vi "Actor Core.vi"(8 "error in":errorcluster, 11 "BrowerController in":refnum<class "BrowerController.lvclass">) -> (0 "error out":errorcluster, 3 "Actor out":refnum<class "Actor.lvclass">)   [LabVIEW 2015, in "BrowerController.lvclass"]
doc: "(<B>Filename</B>: Actor Framework.lvlib:Actor.lvclass:Actor Core.vi)\n\nReceives messages to the actor, reacts to them, and initiates any error handling that may shut the actor down.\n\nDescendant classes may override this VI to append parallel tasks for the actor to complete while it handles messages. Overrides use the Call Parent Method node."
uses:
  BrowerController.lvclass
  <vilib>/ActorFramework/Actor/Actor.lvclass
  Models/BrowerShortcut/BrowerShortcut.lvclass
  Type Definition/Brower UI Refs.ctl
  Models/BrowerTree/BrowerTree.lvclass
  Models/BrowerComponent/BrowerComposite/BrowerComposite.lvclass
  BrowerController.lvclass/BrowerController.ctl
  <vilib>/ActorFramework/Actor/Actor.lvclass/Actor.ctl
  <vilib>/ActorFramework/Message Enqueuer/Message Enqueuer.lvclass/Message Enqueuer.ctl
  Models/BrowerTree/Type Definition/Symbol Index.ctl
  Models/BrowerBuilder/ProjectBuilder/ProjectBuilder.lvclass
  Messages/Add BrowerComponent_Msg/Add BrowerComponent_Msg.lvclass/Add BrowerComponent_Msg.ctl
  Messages/ImportProject_Msg/ImportProject_Msg.lvclass/ImportProject_Msg.ctl
  <vilib>/ActorFramework/Message Enqueuer/Init from Existing Queue.vi
  <vilib>/ActorFramework/Message Enqueuer/Enqueue.vi
  <vilib>/ActorFramework/Message Priority Queue/Priority Enqueue.vi
  <vilib>/ActorFramework/Message Enqueuer/Message Enqueuer.lvclass
  Messages/Add BrowerComponent_Msg/Add BrowerComponent_Msg.lvclass
  Messages/SaveBrowerProject_Msg/SaveBrowerProject_Msg.lvclass
  Messages/ImportProject_Msg/ImportProject_Msg.lvclass
panel:
  out "Value":string
  out "ItemTag":string
  in  "String: BrowerMenu Selection":string
  in  "Tree: Brower":string(tree)
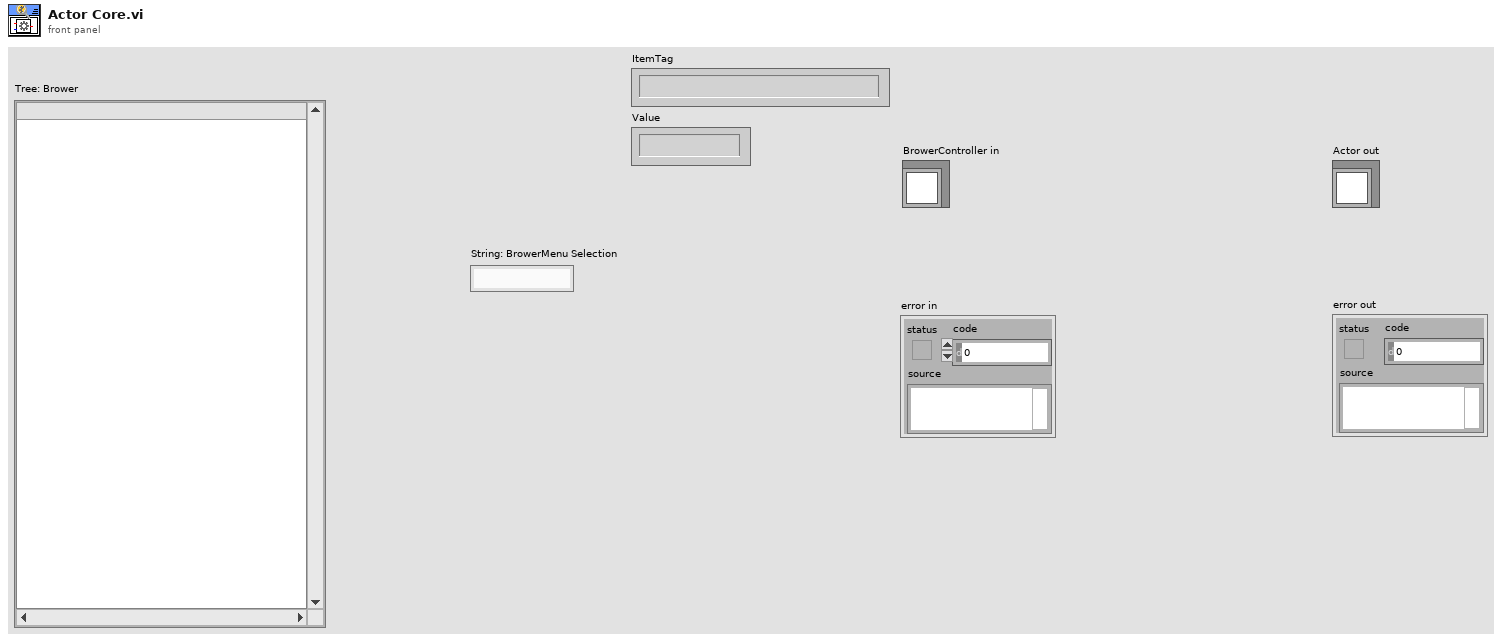
[diagram p1: front panel]
types:
  T1 = typedef "BrowerController.lvclass/Brower UI Refs.ctl" = cluster{"BrowerTree Ref":refnum<vi>, "BrowerMenu Selection(\"\")":refnum<vi>, "VI Refnum":refnum<vi>}
  T2 = typedef "BrowerTree.lvclass/Symbol Index.ctl" = enum16{"PC", "Project", "Module", "DebugTask", "Communication"}
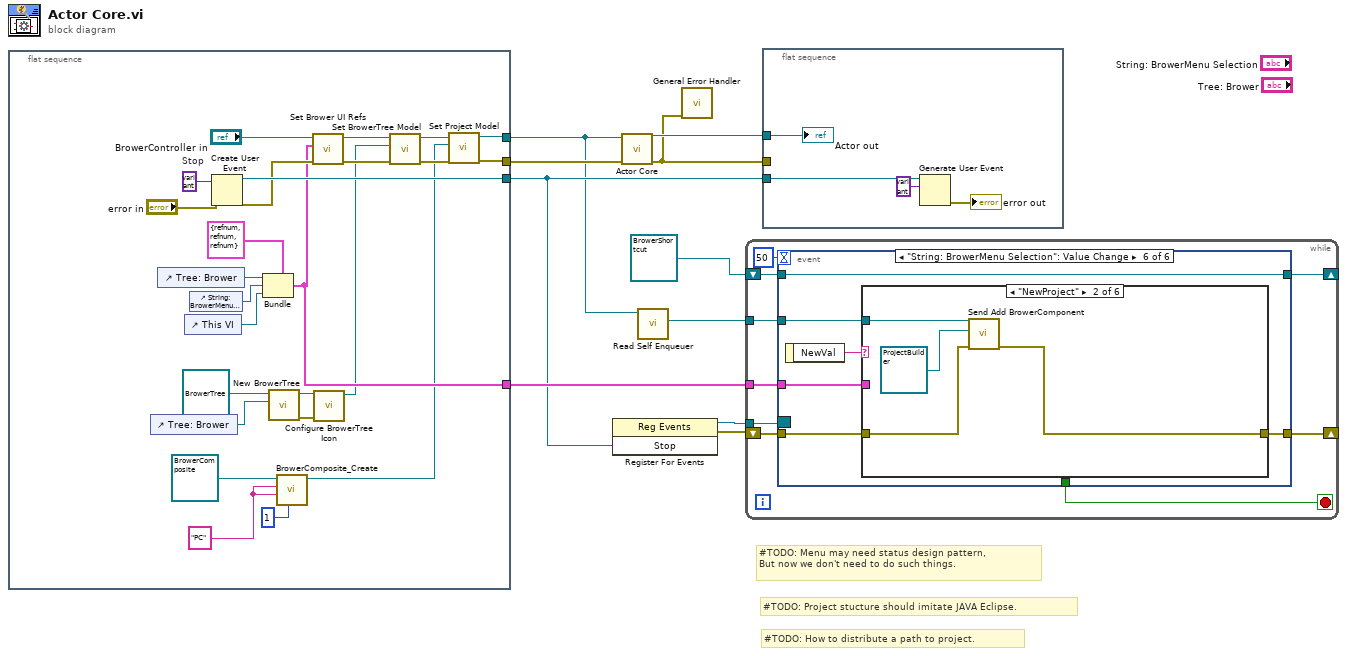
[diagram p0: block diagram]
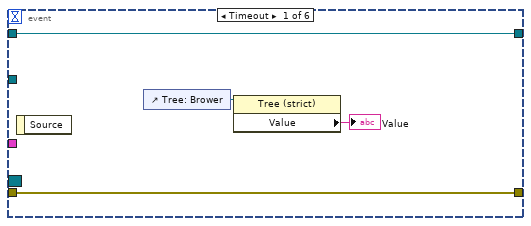
[diagram p2: hidden frame]
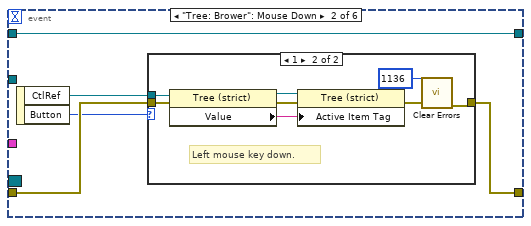
[diagram p3: hidden frame]
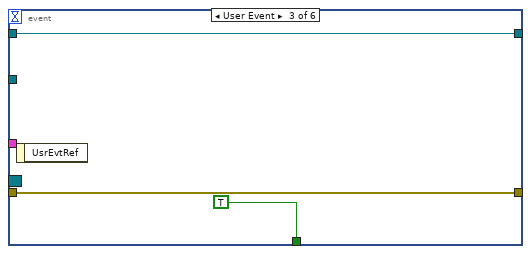
[diagram p5: hidden frame]
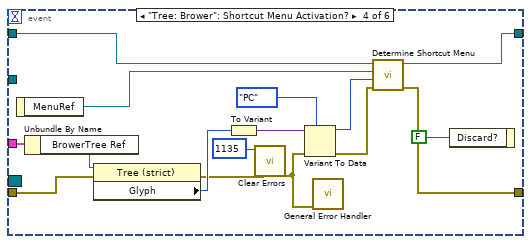
[diagram p6: hidden frame]
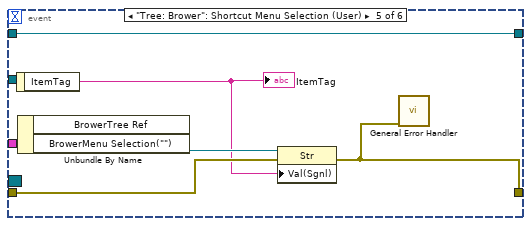
[diagram p7: hidden frame]
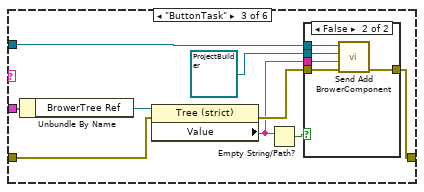
[diagram p9: hidden frame]
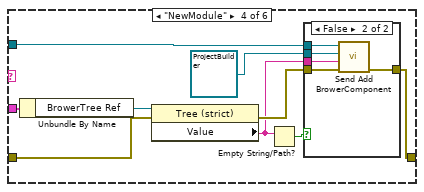
[diagram p11: hidden frame]
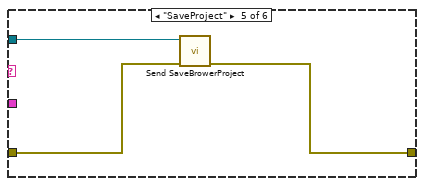
[diagram p13: hidden frame]
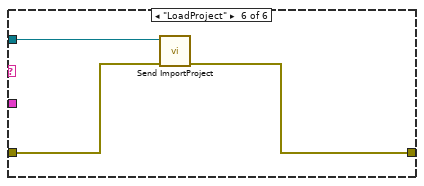
[diagram p14: hidden frame]
diagram:
  # "#TODO: How to distribute a path to project."
  # "#TODO: Project stucture should imitate JAVA Eclipse."
  # "#TODO: Menu may need status design pattern, \nBut now we don't need to do such things."
  n1 = flat-sequence {
    tunnel: [w16] -> w1
    tunnel: [w34] -> w4
    tunnel: [w15] -> w8
    tunnel: [w24] -> w6
    frame #0 {
      w11 = "PC" ("ComponentName")
      w35 = variant  # Stop
      n2 = control-ref of="Tree: Brower"() -> (w27:refnum<vi>)
      n3 = control-ref of="Tree: Brower"() -> (w30:refnum<vi>)
      n4 = control-ref of="This VI"() -> (w23:refnum<vi>)
      n5 = control-ref of="String: BrowerMenu Selection"() -> (w22:refnum<vi>)
      n6 = Create User Event(user event datatype=w35, error in="error in") -> (user event=w34:refnum<user-event>, error out=w29:errorcluster)
      n7 = Bundle(cluster=T1 {"BrowerTree Ref"=refnum, "BrowerMenu Selection(\"\")"=refnum, "VI Refnum"=refnum} ("Brower UI Refs"), "BrowerTree Ref"=w30, "BrowerMenu Selection(\"\")"=w22, "VI Refnum"=w23) -> (w24:T1)
      n8 = call "New BrowerTree.vi"("Tree Refnum"=w27, "BrowerTree in"=refnum<class "BrowerTree.lvclass"> refnum) -> ("error out"=w20:errorcluster, "BrowerTree out"=w21:refnum<class "BrowerTree.lvclass">)  [unwired: 8 in]
      n9 = call "BrowerComposite_Create.vi"("SymbolIndex"=1, "ComponentName"=w11, "ComponentID"=w11, "reference in"=refnum<class "BrowerComposite.lvclass"> refnum) -> ("reference out"=w12:refnum<class "BrowerComposite.lvclass">)  [unwired: 6 in, 1 out]
      n10 = call "Set Brower UI Refs.vi"("error in (no error)"=w29, "Brower UI Refs"=w24, "BrowerController in"="BrowerController in") -> ("error out"=w25:errorcluster, "BrowerController out"=w26:refnum<class "BrowerController.lvclass">)  [unwired: 7 in]
      n11 = call "Configure BrowerTree Icon.vi"("error in (no error)"=w20, "BrowerTree in"=w21) -> ("BrowerTree out"=w19:refnum<class "BrowerTree.lvclass">)  [unwired: 8 in, 1 out]
      n12 = call "Set BrowerTree Model.vi"("error in (no error)"=w25, "BrowerTree.lvclass"=w19, "BrowerController in"=w26) -> ("error out"=w17:errorcluster, "BrowerController out"=w18:refnum<class "BrowerController.lvclass">)  [unwired: 7 in]
      n13 = call "Set Project Model.vi"("error in (no error)"=w17, "Project.lvclass"=w12, "BrowerController in"=w18) -> ("error out"=w15:errorcluster, "BrowerController out"=w16:refnum<class "BrowerController.lvclass">)  [unwired: 7 in]
    }
  }
  n14 = register-events(w4) -> (reference out=w9:refnum<event-registration>, error out=w5:errorcluster)  [unwired: 2 in]
  n15 = call-parent "Actor Core.vi"("error in"=w8, "Actor in"=w1) -> ("error out"=w2:errorcluster, "Actor out"=w10:refnum<class "Actor.lvclass">)  [unwired: 8 in]
  n16 = call <vilib>:"Read Self Enqueuer.vi"("Actor"=w1) -> ("Self Enqueuer"=w3:refnum<class "Message Enqueuer.lvclass">)  [unwired: 10 in]
  n17 = call <vilib>:"General Error Handler.vi"("error in (no error)"=w2) -> ()  [unwired: 10 in, 5 out]
  n18 = while {
    tunnel: w9 -> [w44]
    shift-right: [w38] -> _
    shift-left: refnum<class "BrowerShortcut.lvclass"> refnum ("BrowerShortcut.lvclass") -> [w42]
    tunnel: w6 -> [w41]
    shift-right: [w39] -> _
    shift-left: w5 -> [w40]
    tunnel: w3 -> [w37]
    stop <- w43 stop-if-true
    n19 = event shown="[5] \"String: BrowerMenu Selection\": Value Change" {
      selector: w44 -> [_ _ _ _ _ _]
      dyn-events: _ -> [_ _ _ _ _ _]
      timeout: 50 -> [_ _ _ _ _ _]
      tunnel: [_ _ TRUE _ _ _] -> w43
      tunnel: w42 -> [w48 w53 w64 w81 w87 w93]
      tunnel: w41 -> [_ _ _ w79 w86 w88]
      tunnel: w40 -> [w47 w50 w63 w77 w84 w92]
      tunnel: [w47 w52 w63 w74 w82 w89] -> w39
      tunnel: [w48 w53 w64 w76 w87 w93] -> w38
      tunnel: w37 -> [_ _ _ _ _ w90]
      event Timeout {
        n20 = event-data() -> ()  [unwired: 1 in, 1 out]
        n21 = control-ref of="Tree: Brower"() -> (w46:refnum<vi>)
        n22 = property class="Tree (strict)"(reference=w46) -> ("Value"=→"Value":string)  [unwired: 1 in, 2 out]
      }
      event "Tree: Brower": Mouse Down {
        n23 = event-data() -> ("CtlRef"=w51:refnum<vi>, "Button"=w49:u16)  [unwired: 1 in]
        n24 = case shown="1" w49 {
          tunnel: [w54 w56] -> w52
          tunnel: w51 -> [_ w62]
          tunnel: w50 -> [w54 w61]
          frame 0, Default {
          }
          frame 1 {
            # "Left mouse key down."
            n25 = property class="Tree (strict)"(reference=w62, error in=w61) -> (reference out=w58:refnum<vi>, error out=w59:errorcluster, "Value"=w60:string)
            n26 = property class="Tree (strict)"(reference=w58, error in=w59, "Active Item Tag"=w60) -> (error out=w57:errorcluster)  [unwired: 1 out]
            n27 = call <vilib>:"Clear Errors.vi"("error in (no error)"=w57, "specific error code to clear (0: all)"=1136) -> ("error out"=w56:errorcluster)  [unwired: 4 in, 1 out]
          }
        }
      }
      event User Event {
        n28 = event-data() -> ()  [unwired: 1 in, 1 out]
      }
      event "Tree: Brower": Shortcut Menu Activation? {
        n29 = event-data() -> ("MenuRef"=w80:refnum<k9>)  [unwired: 1 in]
        n30 = Unbundle By Name(w79) -> ("BrowerTree Ref"=w78:refnum<vi>)
        n31 = property class="Tree (strict)"(reference=w78, error in=w77) -> (error out=w68:errorcluster, "Glyph"=w73:i32)  [unwired: 1 out]
        n32 = To Variant(anything=w73) -> (Variant=w72:variant)
        n33 = call <vilib>:"Clear Errors.vi"("error in (no error)"=w68, "specific error code to clear (0: all)"=1135) -> ("error out"=w66:errorcluster)  [unwired: 4 in, 1 out]
        n34 = Variant To Data(error in=w66, type=Symbol_Index."PC" ("SymbolIndex"), Variant=w72) -> (data=w70:T2, error out=w69:errorcluster)
        n35 = call <vilib>:"General Error Handler.vi"("error in (no error)"=w66) -> ()  [unwired: 10 in, 5 out]
        n36 = call "Determine Shortcut Menu.vi"("error in (no error)"=w69, "SymbolIndex"=w70, "Menu Refnum"=w80, "BrowerShortcut in"=w81) -> ("error out"=w74:errorcluster, "BrowerShortcut out"=w76:refnum<class "BrowerShortcut.lvclass">)  [unwired: 6 in]
        n37 = event-data("Discard?"=FALSE) -> ()  [unwired: 1 in, 1 out]
      }
      event "Tree: Brower": Shortcut Menu Selection (User) {
        n38 = event-data() -> ("ItemTag"=w83:string)  [unwired: 1 in]
        "ItemTag" <- w83
        n39 = Unbundle By Name(w86) -> ("BrowerMenu Selection(\"\")"=w85:refnum<vi>)  [unwired: 1 out]
        n40 = property class="Str"(reference=w85, error in=w84, "Val(Sgnl)"=w83) -> (error out=w82:errorcluster)  [unwired: 1 out]
        n41 = call <vilib>:"General Error Handler.vi"("error in (no error)"=w82) -> ()  [unwired: 10 in, 5 out]
      }
      event "String: BrowerMenu Selection": Value Change {
        n42 = event-data() -> ("NewVal"=w91:string)  [unwired: 1 in]
        n43 = case shown="\"NewProject\"" w91 {
          tunnel: w92 -> [w94 w96 w104 w119 w130 w133]
          tunnel: w90 -> [_ w98 w107 w122 w131 w134]
          tunnel: [w94 w95 w101 w116 w129 w132] -> w89
          tunnel: w88 -> [_ _ w106 w121 _ _]
          frame Default {
          }
          frame "NewProject" {
            n44 = call "Send Add BrowerComponent.vi"("error in (no error)"=w96, "Builder"=refnum<class "ProjectBuilder.lvclass"> refnum ("ProjectBuilder"), "Message Enqueuer"=w98) -> ("error out"=w95:errorcluster)  [unwired: 7 in, 1 out]
          }
          frame "ButtonTask" {
            n45 = Unbundle By Name(w106) -> ("BrowerTree Ref"=w105:refnum<vi>)
            n46 = property class="Tree (strict)"(reference=w105, error in=w104) -> (error out=w102:errorcluster, "Value"=w100:string)  [unwired: 1 out]
            n47 = Empty String/Path?(string/path=w100) -> (empty?=w99:bool)
            n48 = case shown="False" w99 {
              tunnel: w107 -> [_ w113]
              tunnel: w100 -> [_ w112]
              tunnel: refnum<class "ProjectBuilder.lvclass"> refnum ("ProjectBuilder") -> [_ w111]
              tunnel: w102 -> [w108 w110]
              tunnel: [w108 w109] -> w101
              frame True {
              }
              frame False {
                n49 = call "Send Add BrowerComponent.vi"("error in (no error)"=w110, "Parent Tag(\"\")"=w112, "Builder"=w111, "Message Enqueuer"=w113) -> ("error out"=w109:errorcluster)  [unwired: 6 in, 1 out]
              }
            }
          }
          frame "NewModule" {
            n50 = Unbundle By Name(w121) -> ("BrowerTree Ref"=w120:refnum<vi>)
            n51 = property class="Tree (strict)"(reference=w120, error in=w119) -> (error out=w117:errorcluster, "Value"=w115:string)  [unwired: 1 out]
            n52 = Empty String/Path?(string/path=w115) -> (empty?=w114:bool)
            n53 = case shown="False" w114 {
              tunnel: w122 -> [_ w128]
              tunnel: w115 -> [_ w127]
              tunnel: refnum<class "ProjectBuilder.lvclass"> refnum ("ProjectBuilder") -> [_ w126]
              tunnel: w117 -> [w123 w125]
              tunnel: [w123 w124] -> w116
              frame True {
              }
              frame False {
                n54 = call "Send Add BrowerComponent.vi"("error in (no error)"=w125, "Parent Tag(\"\")"=w127, "Builder"=w126, "Message Enqueuer"=w128) -> ("error out"=w124:errorcluster)  [unwired: 6 in, 1 out]
              }
            }
          }
          frame "SaveProject" {
            n55 = call "Send SaveBrowerProject.vi"("error in (no error)"=w130, "Message Enqueuer"=w131) -> ("error out"=w129:errorcluster)  [unwired: 8 in, 1 out]
          }
          frame "LoadProject" {
            n56 = call "Send ImportProject.vi"("error in (no error)"=w133, "Message Enqueuer"=w134) -> ("error out"=w132:errorcluster)  [unwired: 8 in, 1 out]
          }
        }
      }
    }
  }
  n57 = flat-sequence {
    tunnel: w10 -> [w138]
    tunnel: w2 -> [_]
    tunnel: w4 -> [w137]
    frame #0 {
      n58 = Generate User Event(user event=w137, event data cluster=variant ("event data")) -> (error out=→"error out":errorcluster)  [unwired: 2 in, 1 out]
      "Actor out" <- w138
    }
  }
